vi "Set Sub Panel Msg.vi"(8 "error in (no error)":errorcluster, 10 "Sub Panel Msg":refnum<vi>, 11 "Msg in":refnum<class "Msg.lvclass">) -> (0 "error out":errorcluster, 3 "Msg out":refnum<class "Msg.lvclass">)   [LabVIEW 2020, in "Msg.lvlib" / "Msg.lvclass"]
uses:
  Msg.lvclass
  Msg.lvclass/Msg.ctl
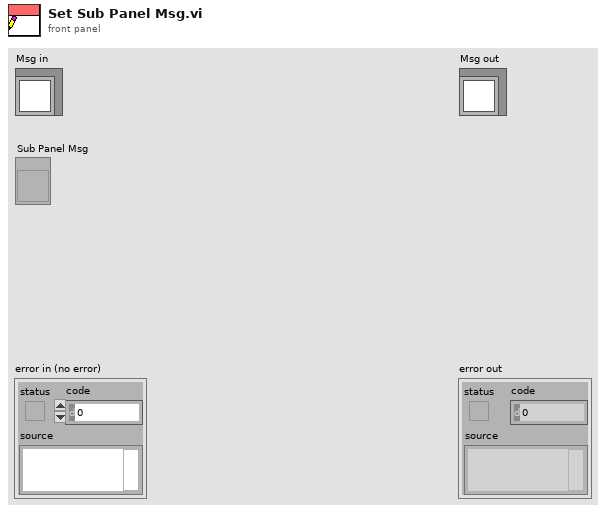
[diagram p1: front panel]
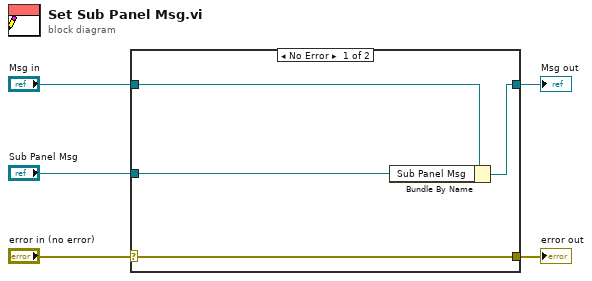
[diagram p0: block diagram]
diagram:
  n1 = case shown="No Error" "error in (no error)" {
    selector: "error in (no error)" -> [w9 w10]
    tunnel: [w9 w10] -> w4
    tunnel: [w7 w11] -> w2
    tunnel: "Msg in" -> [w8 w11]
    tunnel: "Sub Panel Msg" -> [w6 _]
    frame No Error {
      n2 = Bundle By Name(cluster=w8, "Sub Panel Msg"=w6) -> (w7:refnum<class "Msg.lvclass">)
    }
    frame Error {
    }
  }
  "error out" <- w4
  "Msg out" <- w2
